vi "String operations 2.vi"() -> ()   [LabVIEW 2020]
panel:
  out "Output str":string
  in  "Contact":i64
  in  "Age":u8
  in  "Name":string
  out "Output str":string
  in  "replace str":string
  in  "search str":string
  in  "Input str":string
  out "Str Ind 2":string
  in  "Str ctrl 2":string
  out "Str Ind":string
  in  "Str ctrl":string="hi yaar\n"
  # "String Operations 2"
  # "Functions  applied:\n(1) RC -> Data operations\n     ->make current value \n     default\n(2) RC -> Update value \n      while typing"
  # "Functions  applied:\n(1) RC -> '\\' codes display"
  # "Functions  applied:\n(1) RC -> password \n     display"
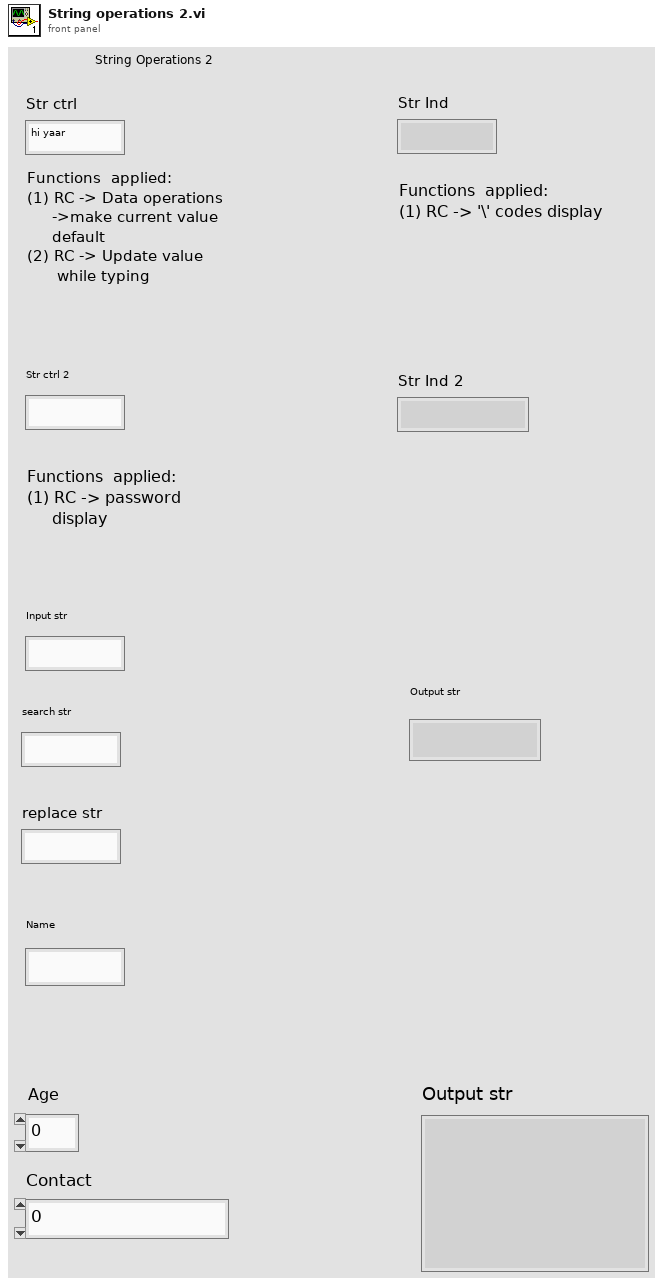
[diagram p1: front panel]
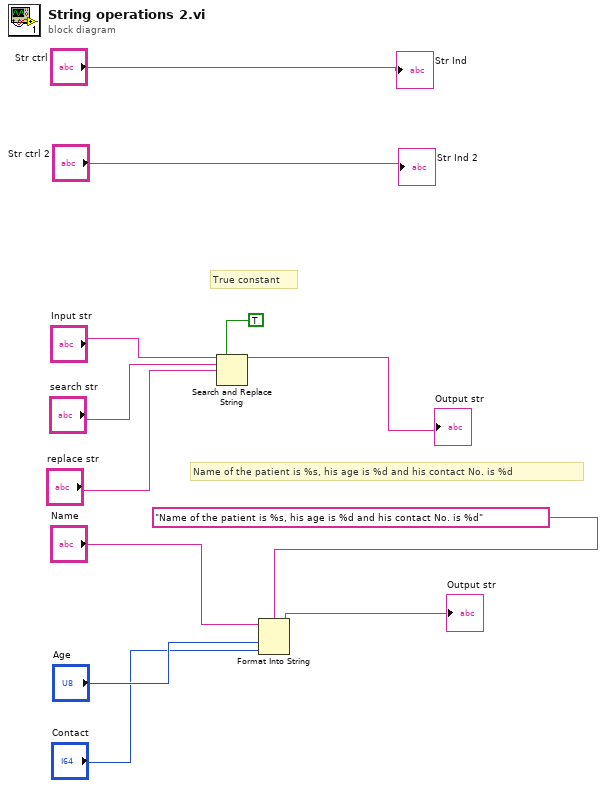
[diagram p0: block diagram]
diagram:
  # "Name of the patient is %s, his age is %d and his contact No. is %d"
  # "True constant"
  n1 = Search and Replace String(replace all?=TRUE, input string="Input str", search string="search str", replace string="replace str") -> (result string=→"Output str":string)  [unwired: 4 in, 3 out]
  n2 = Format Into String(format string="Name of the patient is %s, his age is %d and his contact No. is %d", initial string="Name", "Age", "Contact") -> (resulting string=→"Output str":string)  [unwired: 1 in, 1 out]
  "Str Ind" <- "Str ctrl"
  "Str Ind 2" <- "Str ctrl 2"
